vi "Read ADU Packet.vi"(8 "error in":errorcluster, 10 "protocol layer":refnum<class "Network Protocol.lvclass">, 11 "RTU transmission data unit in":refnum<class "RTU Data Unit.lvclass">) -> (0 "error out":errorcluster, 1 "modbus data unit":refnum<class "Modbus Data Unit.lvclass">, 2 "protocol layer out":refnum<class "Network Protocol.lvclass">, 3 "RTU transmission data unit out":refnum<class "RTU Data Unit.lvclass">, 5 "PDU Valid?":bool)   [LabVIEW 2013, in "Modbus Library - Advance.lvlib" / "RTU Data Unit.lvclass"]
doc: "This uses the protocol layer to read a modbus packet off of the bus, wrapped in the RTU transmission data unit."
uses:
  RTU Data Unit.lvclass
  Modbus Data Unit/Modbus Data Unit.lvclass
  Network Protocol/Network Protocol.lvclass
  Network Protocol/Network Master/Serial/Serial Master.lvclass
  Network Protocol/Network Slave/Serial/Serial Slave.lvclass
  Network Protocol/Network Master/Serial/Serial Master.lvclass/Serial Master.ctl
  Network Protocol/Network Slave/Serial/Serial Slave.lvclass/Serial Slave.ctl
  Transmission Data Unit.lvclass/Transmission Data Unit.ctl
  RTU Data Unit.lvclass/RTU Data Unit.ctl
  Serial Interface/Serial Data Unit.lvclass/Serial Data Unit.ctl
  Modbus Data Unit/Modbus Data Unit.lvclass/Modbus Data Unit.ctl
  Serial Interface/Serial acquisition states.ctl
  buffer element.ctl
  <vilib>/ErrorRing/Error Ring.xnode
  Serial Interface/Serial Data Unit.lvclass
  Transmission Data Unit.lvclass
  Serial Shared Components/Serial Shared Components.lvlib
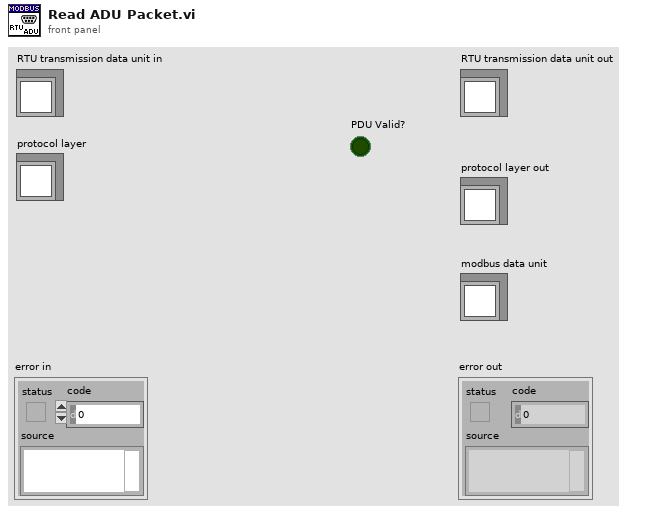
[diagram p1: front panel]
types:
  T1 = typedef "Modbus Library - Advance.lvlib/RTU Data Unit.lvclass/buffer element.ctl" = cluster{"data":u8[], "packets contained":i32}
  T2 = typedef "Modbus Library - Advance.lvlib/Serial Data Unit.lvclass/Serial acquisition states.ctl" = enum16{"Wait for frame", "Check for validity"}
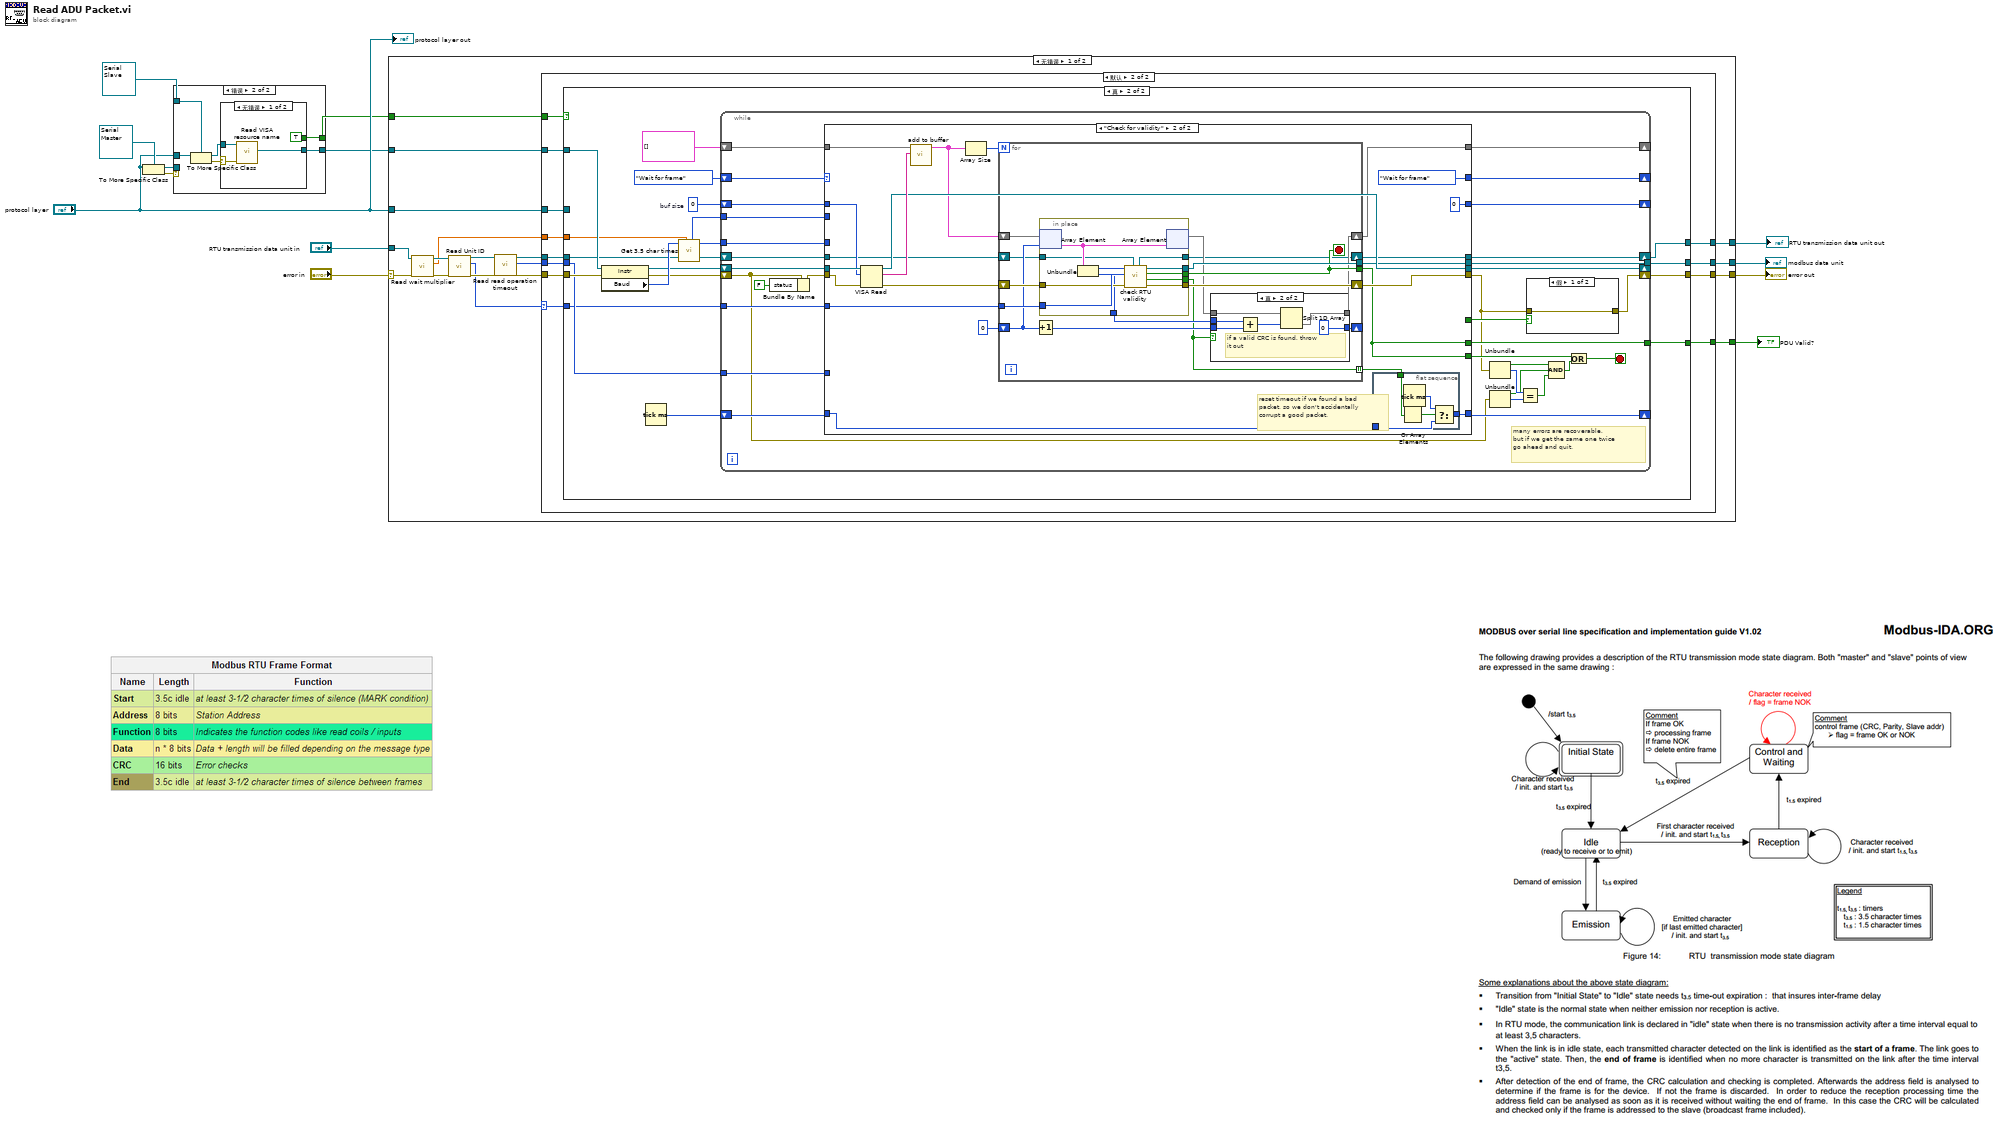
[diagram p0: block diagram]
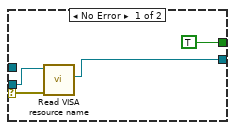
[diagram p2: hidden frame]
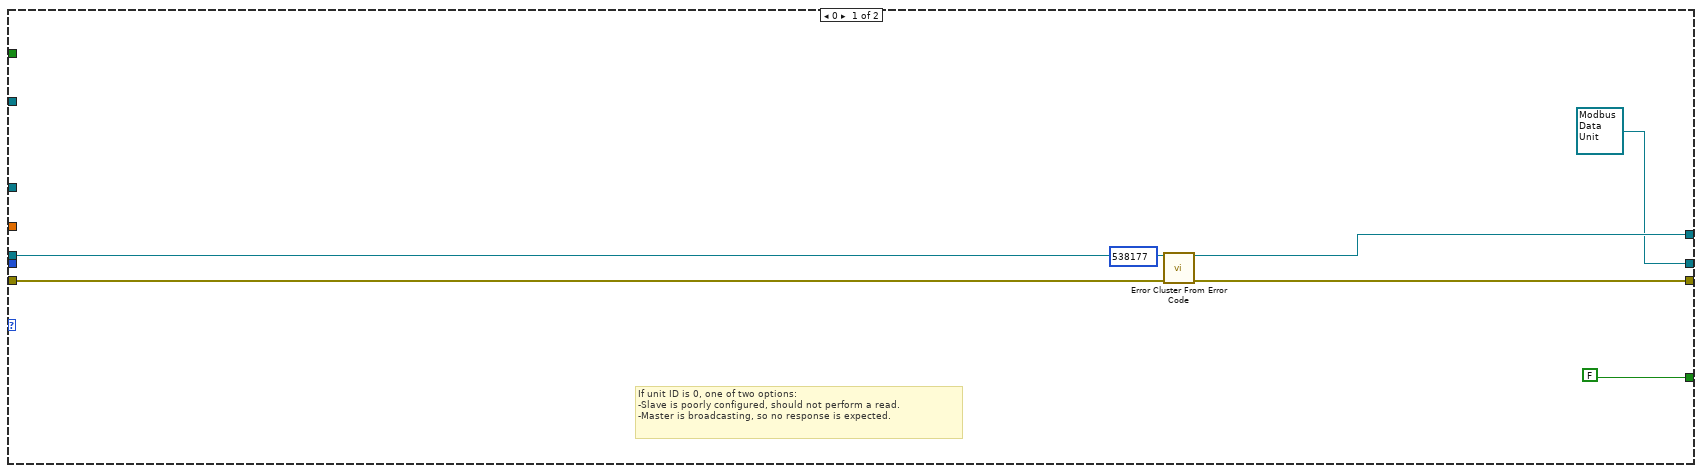
[diagram p4: hidden frame]
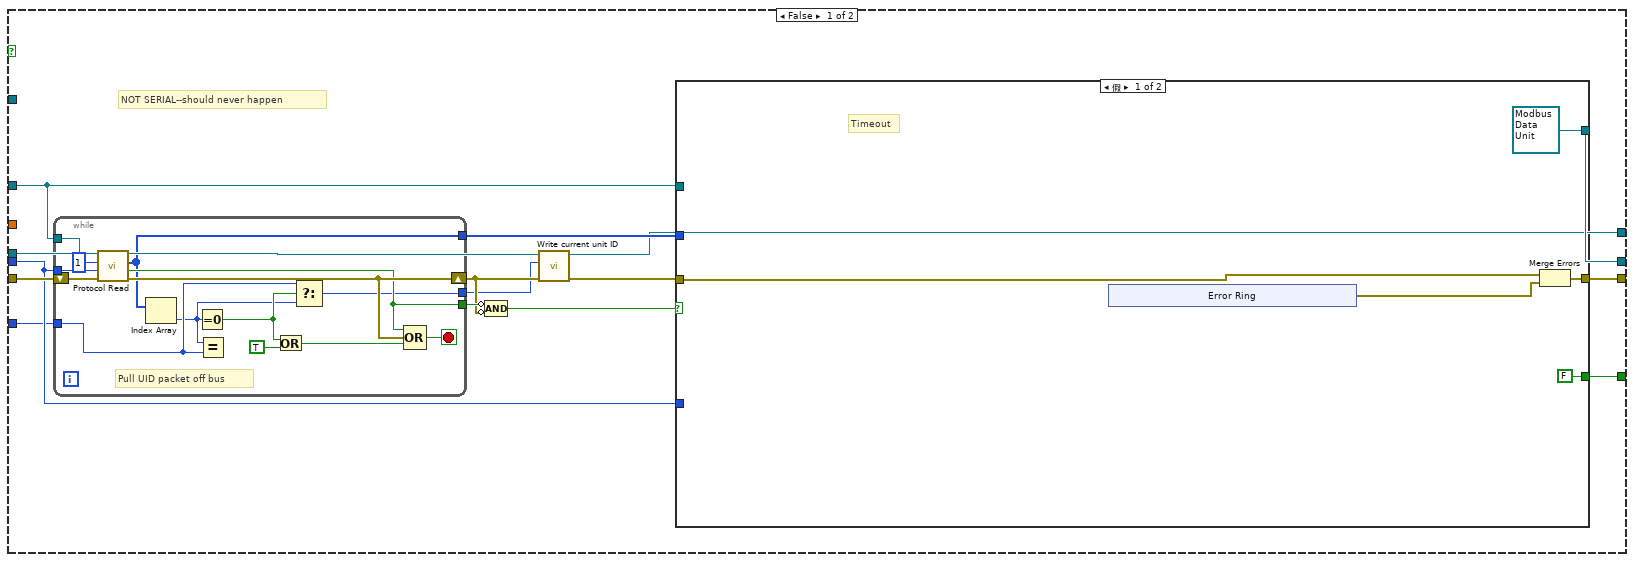
[diagram p5: hidden frame]
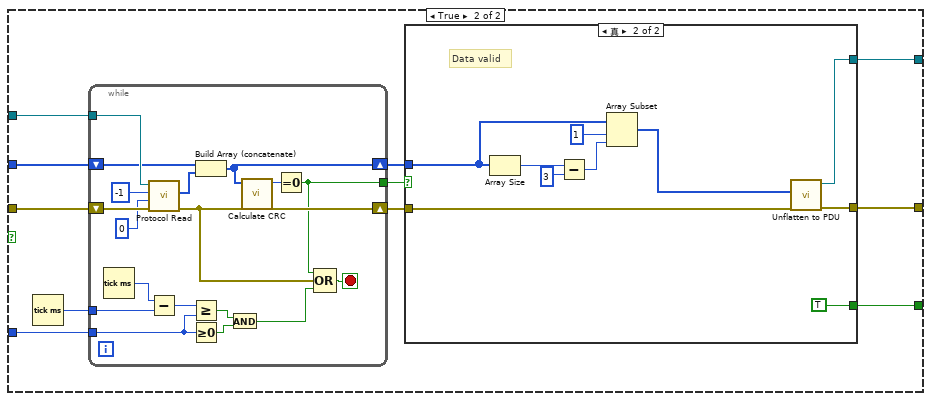
[diagram p6: hidden frame]
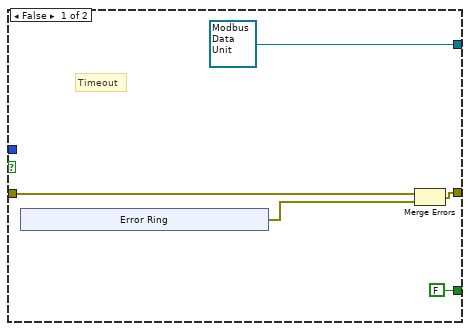
[diagram p7: hidden frame]
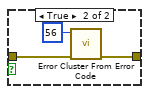
[diagram p8: hidden frame]
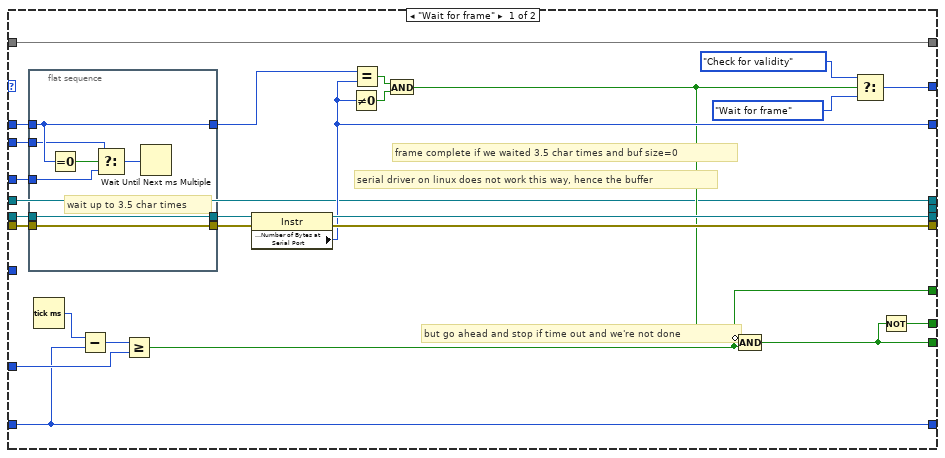
[diagram p9: hidden frame]
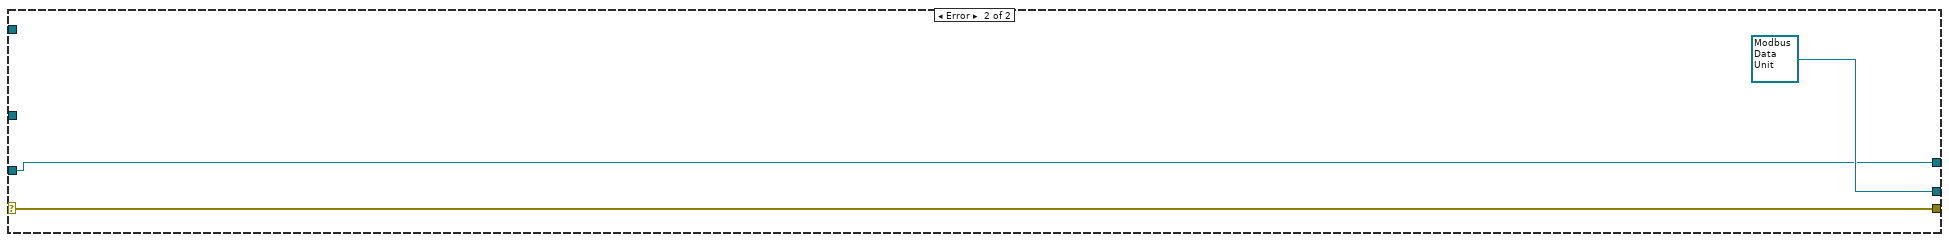
[diagram p11: hidden frame]
diagram:
  n1 = To More Specific Class(target class=refnum<class "Serial Master.lvclass"> refnum ("Serial Master"), reference="protocol layer") -> (specific class reference=w2:refnum<class "Serial Master.lvclass">, error out=w6:errorcluster)  [unwired: 1 in]
  n2 = case shown="错误" w6 {
    selector: w6 -> [w16 _]
    tunnel: "protocol layer" -> [_ w23]
    tunnel: [TRUE w21] -> w4
    tunnel: refnum<class "Serial Slave.lvclass"> refnum ("Serial Slave") -> [_ w20]
    tunnel: [w14 w18] -> w1
    tunnel: w2 -> [w15 _]
    frame No Error {
      n3 = call "Read VISA resource name.vi"("error in (no error)"=w16, "Serial Master in"=w15) -> ("VISA resource name"=w14:refnum<visa-resource-name>)  [unwired: 7 in, 2 out]
    }
    frame Error {
      n4 = To More Specific Class(target class=w20, reference=w23) -> (specific class reference=w19:refnum<class "Serial Slave.lvclass">, error out=w22:errorcluster)  [unwired: 1 in]
      n5 = case shown="无错误" w22 {
        selector: w22 -> [w26 _]
        tunnel: [TRUE _] -> w21
        tunnel: w19 -> [w25 _]
        tunnel: [w24 _] -> w18
        frame No Error {
          n6 = call "Read VISA resource name.vi"("error in (no error)"=w26, "Serial Slave in"=w25) -> ("VISA resource name"=w24:refnum<visa-resource-name>)  [unwired: 7 in, 2 out]
        }
        frame Error {
        }
      }
    }
  }
  n7 = case shown="无错误" "error in" {
    selector: "error in" -> [w32 w301]
    tunnel: [w45 w301] -> w12
    tunnel: "RTU transmission data unit in" -> [w28 w299]
    tunnel: "protocol layer" -> [w43 _]
    tunnel: [w44 refnum<class "Modbus Data Unit.lvclass"> refnum ("modbus data unit")] -> w11
    tunnel: [w42 w299] -> w9
    tunnel: [w35 _] -> w8
    tunnel: w4 -> [w34 _]
    tunnel: w1 -> [w33 _]
    frame No Error {
      n8 = call "Read wait multiplier.vi"("error in (no error)"=w32, "RTU Data Unit in"=w28) -> ("error out"=w31:errorcluster, "wait multiplier"=w29:sgl, "RTU Data Unit out"=w30:refnum<class "RTU Data Unit.lvclass">)  [unwired: 7 in]
      n9 = call "Read Unit ID.vi"("error in"=w31, "transmission data unit in"=w30) -> ("error out"=w39:errorcluster, "unit ID"=w37:u8, "transmission data unit out"=w38:refnum<class "RTU Data Unit.lvclass">)  [unwired: 7 in]
      n10 = call "Read read operation timeout.vi"("error in (no error)"=w39, "transmission data unit in"=w38) -> ("error out"=w40:errorcluster, "read operation timeout"=w36:i32, "transmission data unit out"=w41:refnum<class "RTU Data Unit.lvclass">)  [unwired: 7 in]
      n11 = case shown="默认" w37 {
        selector: w37 -> [_ w58]
        tunnel: w40 -> [w51 w63]
        tunnel: [w47 w62] -> w45
        tunnel: [refnum<class "Modbus Data Unit.lvclass"> refnum ("modbus data unit out") w61] -> w44
        tunnel: w43 -> [_ w60]
        tunnel: w36 -> [_ w59]
        tunnel: w41 -> [w50 w56]
        tunnel: [w50 w57] -> w42
        tunnel: [FALSE w55] -> w35
        tunnel: w34 -> [_ w54]
        tunnel: w33 -> [_ w53]
        tunnel: w29 -> [_ w52]
        frame 0 {
          # "If unit ID is 0, one of two options:\n-Slave is poorly configured, should not perform a read.\n-Master is broadcasting, so no response is expected."
          n12 = call <vilib>:"Error Cluster From Error Code.vi"("error in (no error)"=w51, "error code (0)"=538177) -> ("error out"=w47:errorcluster)  [unwired: 7 in]
        }
        frame Default {
          n13 = case shown="真" w54 {
            tunnel: w63 -> [w78 w167]
            tunnel: [w75 w164] -> w62
            tunnel: [w74 w155] -> w61
            tunnel: w60 -> [w73 _]
            tunnel: w59 -> [w71 w159]
            tunnel: w58 -> [w70 w156]
            tunnel: [w69 w150] -> w57
            tunnel: w56 -> [w67 w151]
            tunnel: [w65 w157] -> w55
            tunnel: w53 -> [_ w166]
            tunnel: w52 -> [_ w152]
            frame False {
              # "NOT SERIAL--should never happen"
              n14 = while {
                shift-right: [w146] -> w66
                shift-left: w78 -> [w149]
                tunnel: w71 -> [w144]
                tunnel: w70 -> [w138]
                tunnel: [w142] -> w77
                tunnel: [w141] -> w72
                tunnel: w73 -> [w148]
                tunnel: [w136] -> w64
                stop <- w147 stop-if-true
                # "Pull UID packet off bus"
                n15 = call-dynamic "Protocol Read.vi"("error in"=w149, "timeout"=w144, "bytes to read"=1, "protocol layer in"=w148) -> ("error out"=w146:errorcluster, "timed out?"=w142:bool, "data"=w141:u8[])  [unwired: 4 in, 1 out]
                n16 = Index Array(array=w141) -> (element=w137:u8)  [unwired: 1 in]
                n17 = Equal To 0?(x=w137) -> (x = 0?=w139:bool)
                n18 = Equal?(x=w137, y=w138) -> ()  [unwired: 1 out]
                n19 = Or(x=w139, y=TRUE) -> (x .or. y?=w143:bool)
                n20 = Select(t=w138, s=w139, f=w137) -> (s? t:f=w136:u8)
                n21 = Compound Arithmetic op=OR(w142, w146, w143) -> (w147:bool)
              }
              n22 = Compound Arithmetic op=AND(invert w77, invert w66) -> (w76:bool)
              n23 = call "Write current unit ID.vi"("error in (no error)"=w66, "request unit ID"=w64, "Serial Data Unit in"=w67) -> ("error out"=w68:errorcluster, "Serial Data Unit out"=w69:refnum<class "RTU Data Unit.lvclass">)  [unwired: 7 in]
              n24 = case shown="假" w76 {
                tunnel: w68 -> [w81 w98]
                tunnel: [w82 w90] -> w75
                tunnel: [refnum<class "Modbus Data Unit.lvclass"> refnum ("modbus data unit out") w91] -> w74
                tunnel: w73 -> [_ w94]
                tunnel: w72 -> [_ w95]
                tunnel: w71 -> [_ w96]
                tunnel: [FALSE w88] -> w65
                frame False {
                  # "Timeout"
                  n25 = xnode "Error Ring"() -> ("错误输出"=w83:errorcluster)
                  n26 = Merge Errors(w81, w83) -> (w82:errorcluster)
                }
                frame True {
                  n27 = Tick Count (ms)() -> (millisecond timer value=w97:u32)
                  n28 = while {
                    shift-right: [w121] -> w92
                    shift-left: w98 -> [w127]
                    tunnel: w97 -> [w135]
                    tunnel: w96 -> [w132]
                    shift-right: [w119] -> w89
                    shift-left: w95 -> [w123]
                    tunnel: w94 -> [w126]
                    tunnel: [w118] -> w93
                    stop <- w129 stop-if-true
                    n29 = Tick Count (ms)() -> (millisecond timer value=w134:u32)
                    n30 = call-dynamic "Protocol Read.vi"("error in"=w127, "timeout"=0, "bytes to read"=-1, "protocol layer in"=w126) -> ("error out"=w121:errorcluster, "data"=w122:u8[])  [unwired: 4 in, 2 out]
                    n31 = Subtract(x=w134, y=w135) -> (x-y=w133:u32)
                    n32 = Greater Or Equal?(x=w133, y=w132) -> (x >= y?=w130:bool)
                    n33 = Greater Or Equal To 0?(x=w132) -> (x >= 0?=w131:bool)
                    n34 = Build Array (concatenate)(w123, w122) -> (w119:u8[])
                    n35 = And(x=w130, y=w131) -> (x .and. y?=w128:bool)
                    n36 = call "Calculate CRC.vi"("data"=w119) -> ("CRC-16"=w120:u16)  [unwired: 10 in]
                    n37 = Equal To 0?(x=w120) -> (x = 0?=w118:bool)
                    n38 = Compound Arithmetic op=OR(w118, w121, w128) -> (w129:bool)
                  }
                  n39 = case shown="真" w93 {
                    tunnel: w92 -> [w101 w115]
                    tunnel: [refnum<class "Modbus Data Unit.lvclass"> refnum ("modbus data unit") w116] -> w91
                    tunnel: [w100 w117] -> w90
                    tunnel: w89 -> [_ w109]
                    tunnel: [FALSE TRUE] -> w88
                    frame False {
                      # "Timeout"
                      n40 = xnode "Error Ring"() -> ("错误输出"=w102:errorcluster)
                      n41 = Merge Errors(w101, w102) -> (w100:errorcluster)
                    }
                    frame True {
                      # "Data valid"
                      n42 = Array Size(array=w109) -> (size(s)=w113:i32)
                      n43 = Subtract(x=w113, y=3) -> (x-y=w111:i32)
                      n44 = Array Subset(array=w109, index=1, length=w111) -> (w110:u8[])
                      n45 = call "Unflatten to PDU.vi"("error in"=w115, "modbus data unit data"=w110) -> ("error out"=w117:errorcluster, "modbus data unit out"=w116:refnum<class "Modbus Data Unit.lvclass">)  [unwired: 8 in]
                    }
                  }
                }
              }
            }
            frame True {
              w161 = u32 0  # buf size
              n46 = property class="Instr"(reference=w166, error in=w167) -> (reference out=w163:refnum<visa-resource-name>, error out=w165:errorcluster, "Baud"=w168:u32)
              n47 = Tick Count (ms)() -> (millisecond timer value=w160:u32)
              n48 = call "Get 3.5 char times.vi"("wait multiplier"=w152, "baud rate"=w168) -> ("wait time (ms)"=w158:u32, "initial wait (ms)"=w154:u32)  [unwired: 8 in]
              n49 = while {
                shift-right: [w187] -> w164
                shift-left: w165 -> [w177]
                shift-right: [w193] -> _
                shift-left: w163 -> [w199]
                shift-right: [w192] -> _
                shift-left: Serial_acquisition_states."Wait for frame" ("Serial Acquisition States") -> [w200]
                shift-right: [w194] -> _
                shift-left: w161 -> [w196]
                tunnel: w159 -> [w197]
                tunnel: w158 -> [w195]
                tunnel: [w191] -> w157
                tunnel: w156 -> [w190]
                tunnel: [w189] -> w155
                tunnel: w154 -> [w186]
                shift-right: [w184] -> _
                shift-left: T1[] [] -> [w185]
                shift-right: [w183] -> _
                shift-left: w160 -> [w198]
                shift-right: [w169] -> w150
                shift-left: w151 -> [w170]
                stop <- w180 stop-if-true
                # "many errors are recoverable,\nbut if we get the same one twice\ngo ahead and quit."
                n50 = Bundle By Name(cluster=w177, "status"=FALSE) -> (w182:errorcluster)
                n51 = case shown="\"Check for validity\"" w200 {
                  tunnel: w199 -> [w226 w258]
                  tunnel: w182 -> [w225 w259]
                  tunnel: w198 -> [w206 w241]
                  tunnel: w197 -> [w228 _]
                  tunnel: w196 -> [w223 w257]
                  tunnel: w195 -> [w222 _]
                  tunnel: [w213 u32 0 ("Bytes at Port")] -> w194
                  tunnel: [w210 w242] -> w179
                  tunnel: [w218 w252] -> w178
                  tunnel: [w217 w251] -> w193
                  tunnel: [w214 Serial_acquisition_states."Wait for frame" ("Serial Acquisition States")] -> w192
                  tunnel: [w211 w242] -> w191
                  tunnel: w190 -> [_ w255]
                  tunnel: [_ w249] -> w189
                  tunnel: [w209 _] -> w188
                  tunnel: w186 -> [w208 _]
                  tunnel: w185 -> [w207 w248]
                  tunnel: [w207 w244] -> w184
                  tunnel: [w206 w243] -> w183
                  tunnel: w170 -> [w205 w239]
                  tunnel: [w205 w238] -> w169
                  frame "Wait for frame" {
                    # "serial driver on linux does not work this way, hence the buffer"
                    # "but go ahead and stop if time out and we're not done"
                    # "frame complete if we waited 3.5 char times and buf size=0"
                    n52 = flat-sequence {
                      tunnel: [w237] -> w227
                      tunnel: w226 -> [w237]
                      tunnel: w225 -> [w236]
                      tunnel: [w236] -> w224
                      tunnel: w223 -> [w235]
                      tunnel: [w235] -> w219
                      tunnel: w222 -> [w233]
                      tunnel: w208 -> [w231]
                      frame #0 {
                        # "wait up to 3.5 char times"
                        n53 = Equal To 0?(x=w235) -> (x = 0?=w234:bool)
                        n54 = Select(t=w231, s=w234, f=w233) -> (s? t:f=w232:u32)
                        n55 = Wait Until Next ms Multiple(millisecond multiple=w232) -> ()  [unwired: 1 out]
                      }
                    }
                    n56 = Tick Count (ms)() -> (millisecond timer value=w230:u32)
                    n57 = Subtract(x=w230, y=w206) -> (x-y=w229:u32)
                    n58 = Greater Or Equal?(x=w229, y=w228) -> (x >= y?=w209:bool)
                    n59 = property class="Instr"(reference=w227, error in=w224) -> (reference out=w217:refnum<visa-resource-name>, error out=w218:errorcluster, "Serial Settings:Number of Bytes at Serial Port"=w213:u32)
                    n60 = Not Equal To 0?(x=w213) -> (x != 0?=w221:bool)
                    n61 = Equal?(x=w219, y=w213) -> (x = y?=w220:bool)
                    n62 = And(x=w220, y=w221) -> (x .and. y?=w212:bool)
                    n63 = Compound Arithmetic op=AND(invert w212, w209) -> (w210:bool)
                    n64 = Select(t=Serial_acquisition_states."Check for validity" ("Serial Acquisition States"), s=w212, f=Serial_acquisition_states."Wait for frame" ("Serial Acquisition States")) -> (s? t:f=w214:T2)
                    n65 = Not(x=w210) -> (.not. x?=w211:bool)
                  }
                  frame "Check for validity" {
                    # "reset timeout if we found a bad\npacket, so we don't accidentally\ncorrupt a good packet."
                    n66 = VISA Read(VISA resource name=w258, byte count=w257, error in (no error)=w259) -> (VISA resource name out=w251:refnum<visa-resource-name>, read buffer=w256:string, error out=w254:errorcluster)  [unwired: 1 out]
                    n67 = call "add to buffer.vi"("read data"=w256, "buffer in"=w248) -> ("buffer out"=w245:T1[])  [unwired: 9 in]
                    n68 = Array Size(array=w245) -> (size(s)=w246:i32)
                    n69 = for {
                      N: w246 -> [_]
                      tunnel: w255 -> [w274]
                      tunnel: [w277] -> w249
                      shift-right: [w278] -> w252
                      shift-left: w254 -> [w279]
                      shift-right: [w269] -> _
                      shift-left: 0 -> [w273]
                      shift-right: [w270] -> w244
                      shift-left: w245 -> [w275]
                      tunnel: [w276] -> w242
                      tunnel: [w267] -> w240 mode=indexing
                      shift-right: [w265] -> w238
                      shift-left: w239 -> [w266]
                      stop <- w276 stop-if-true
                      n70 = Increment(x=w273) -> (x+1=w272:i32)
                      n71 = in-place {
                        in-place-border: w274 -> [w298]
                        in-place-border: w279 -> [w297]
                        in-place-border: [w296] -> w278
                        in-place-border: [w295] -> w277
                        in-place-border: [w294] -> w276
                        in-place-border: [w293] -> w267
                        in-place-border: [w290] -> w268
                        in-place-border: w266 -> [w289]
                        in-place-border: [w288] -> w265
                        n72 = in-place-array #1(w275, w273) -> (w292:T1)
                        n73 = Unbundle(w292) -> ("data"=w291:u8[], "packets contained"=w290:i32)
                        n74 = call "check RTU validity.vi"("RTU transmission data unit in"=w289, "error in (no error)"=w297, "unit ID"=w298, "unsigned byte array"=w291) -> ("error out"=w296:errorcluster, "valid packet"=w293:bool, "valid PDU"=w294:bool, "Modbus Data Unit out"=w295:refnum<class "Modbus Data Unit.lvclass">, "RTU transmission data unit out"=w288:refnum<class "RTU Data Unit.lvclass">)  [unwired: 3 in]
                        n75 = in-place-array #1(w292) -> (w271:T1[])  [unwired: 1 out]
                      }
                      n76 = case shown="真" w267 {
                        tunnel: w271 -> [w281 w287]
                        tunnel: w272 -> [w280 w286]
                        tunnel: [w281 w284] -> w270
                        tunnel: [w280 0] -> w269
                        tunnel: w268 -> [_ w282]
                        frame False {
                        }
                        frame True {
                          # "if a valid CRC is found, throw\nit out"
                          n77 = Add(x=w282, y=w286) -> (x+y=w283:i32)
                          n78 = Split 1D Array(array=w287, index=w283) -> (second subarray=w284:T1[])  [unwired: 1 out]
                        }
                      }
                    }
                    n79 = flat-sequence {
                      tunnel: [w264] -> w243
                      tunnel: w241 -> [w263]
                      tunnel: w240 -> [w261]
                      frame #0 {
                        n80 = Or Array Elements(Boolean array=w261) -> (logical OR=w262:bool)
                        n81 = Tick Count (ms)() -> (millisecond timer value=w260:u32)
                        n82 = Select(t=w260, s=w262, f=w263) -> (s? t:f=w264:u32)
                      }
                    }
                  }
                }
                n83 = Unbundle(w178) -> ("status"=w174:bool, "code"=w175:i32)  [unwired: 1 out]
                n84 = Unbundle(w177) -> ("status"=w173:bool, "code"=w176:i32)  [unwired: 1 out]
                n85 = Equal?(x=w175, y=w176) -> (x = y?=w171:bool)
                n86 = case shown="假" w188 {
                  tunnel: w178 -> [w201 w204]
                  tunnel: [w201 w203] -> w187
                  frame False {
                  }
                  frame True {
                    n87 = call <vilib>:"Error Cluster From Error Code.vi"("error in (no error)"=w204, "error code (0)"=56) -> ("error out"=w203:errorcluster)  [unwired: 7 in]
                  }
                }
                n88 = Compound Arithmetic op=AND(w174, w173, w171) -> (w172:bool)
                n89 = Or(x=w179, y=w172) -> (x .or. y?=w180:bool)
              }
            }
          }
        }
      }
    }
    frame Error {
    }
  }
  "RTU transmission data unit out" <- w9
  "modbus data unit" <- w11
  "error out" <- w12
  "PDU Valid?" <- w8
  "protocol layer out" <- "protocol layer"
